vi "Parse_Imp_Data.vi"(8 "error in (no error)":errorcluster) -> (0 "error out":errorcluster, 3 "Resistance":dbl format="%.6g")   [LabVIEW 2020]
panel:
  out "read buffer":string
  out "Reactance":dbl
  out "EndResist":i32
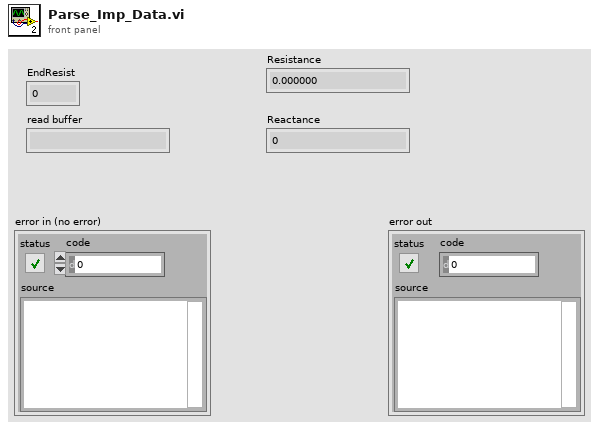
[diagram p1: front panel]
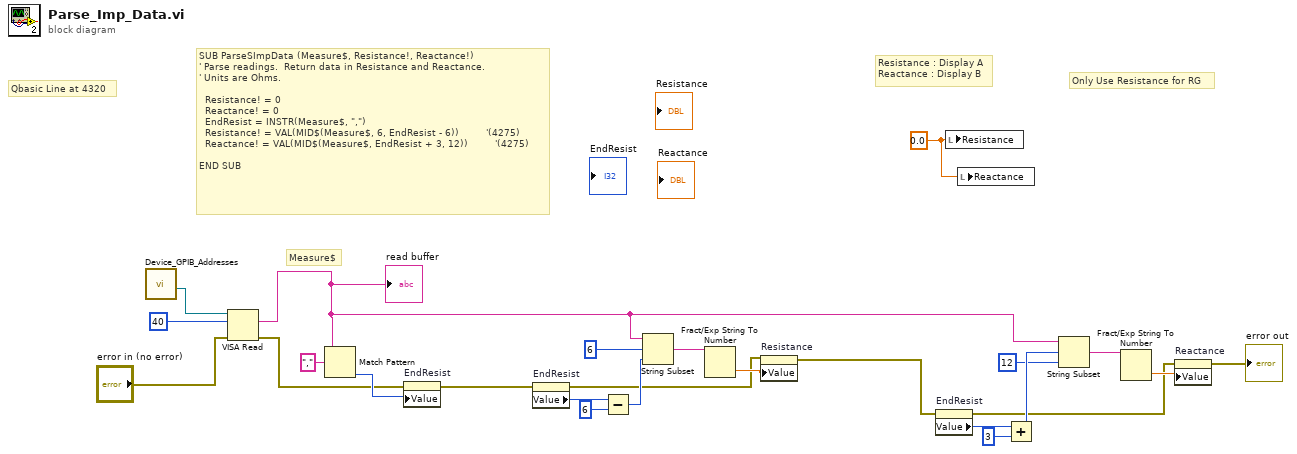
[diagram p0: block diagram]
diagram:
  w6 = 0.0 ("Resistance")
  # "Only Use Resistance for RG"
  # "Resistance : Display A\nReactance : Display B"
  # "Measure$"
  # "Qbasic Line at 4320"
  # "SUB ParseSImpData (Measure$, Resistance!, Reactance!)\n' Parse readings.  Return data in Resistance and Reactance.\n' Units are Ohms.\n\n  Resistance! = 0\n  Reactance! = 0\n  EndResist = INSTR(Measure$, \",\")\n  Resistance! = VAL(MID$(Measure$, 6, EndResist - 6))         '(4275)\n  Reactance! = VAL(MID$(Measure$, EndResist + 3, 12))         '(4275)\n\nEND SUB"
  n1 = call "Device_GPIB_Addresses.vi"() -> ("HP 4275A Address"=w24:refnum<visa-resource-name>)  [unwired: 9 in, 2 out]
  n2 = VISA Read(VISA resource name=w24, byte count=40, error in (no error)="error in (no error)") -> (read buffer=w12:string, error out=w20:errorcluster)  [unwired: 2 out]
  "read buffer" <- w12
  n3 = Match Pattern(string=w12, regular expression=",") -> (offset past match=w21:i32)  [unwired: 1 in, 3 out]
  n4 = property on="EndResist" class="DigNum (strict)"(error in=w20, "Value"=w21) -> (error out=w4:errorcluster)  [unwired: 1 in, 1 out]
  n5 = property on="EndResist" class="DigNum (strict)"(error in=w4) -> (error out=w3:errorcluster, "Value"=w18:i32)  [unwired: 1 in, 1 out]
  n6 = Subtract(x=w18, y=6) -> (x-y=w16:i32)
  n7 = String Subset(string=w12, offset (0)=6, length (rest)=w16) -> (substring=w15:string)
  n8 = Fract/Exp String To Number(string=w15) -> (number=w14:dbl)  [unwired: 3 in, 1 out]
  n9 = property on="Resistance" class="DigNum (strict)"(error in=w3, "Value"=w14) -> (error out=w2:errorcluster)  [unwired: 1 in, 1 out]
  n10 = property on="EndResist" class="DigNum (strict)"(error in=w2) -> (error out=w1:errorcluster, "Value"=w10:i32)  [unwired: 1 in, 1 out]
  n11 = local write "Resistance"(w6) -> ()
  n12 = local write "Reactance"(w6) -> ()
  n13 = Add(x=w10, y=3) -> (x+y=w9:i32)
  n14 = String Subset(string=w12, offset (0)=w9, length (rest)=12 ("length (rest)")) -> (substring=w13:string)
  n15 = Fract/Exp String To Number(string=w13) -> (number=w7:dbl)  [unwired: 3 in, 1 out]
  n16 = property on="Reactance" class="DigNum (strict)"(error in=w1, "Value"=w7) -> (error out=→"error out":errorcluster)  [unwired: 1 in, 1 out]
